vi "Lock VI.vi"(11 "文件路径":path) -> ()   [LabVIEW 2012]
panel:
  in  "密码":string="Jazz@0422g"
  out "滑动杆":i32(slide) scale=0.0..50.0
  out "All Files in Dir":path[](array[path]) caption="目录中的所有文件"
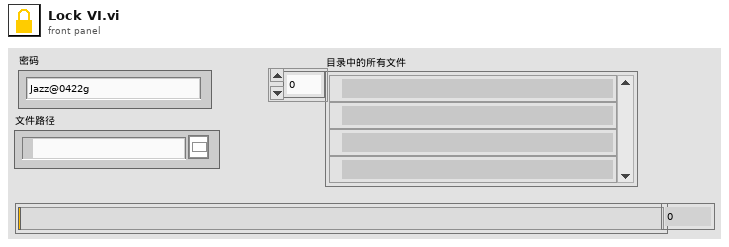
[diagram p1: front panel]
types:
  T1 = enum32{"invalid lock state", "Not Locked", "Locked (No Password)", "Password-protected"}
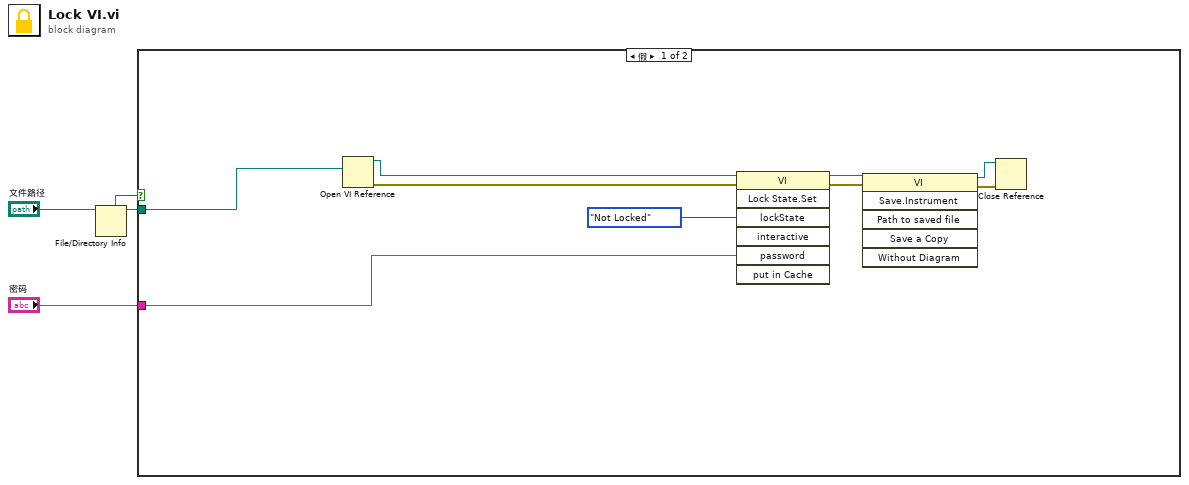
[diagram p0: block diagram]
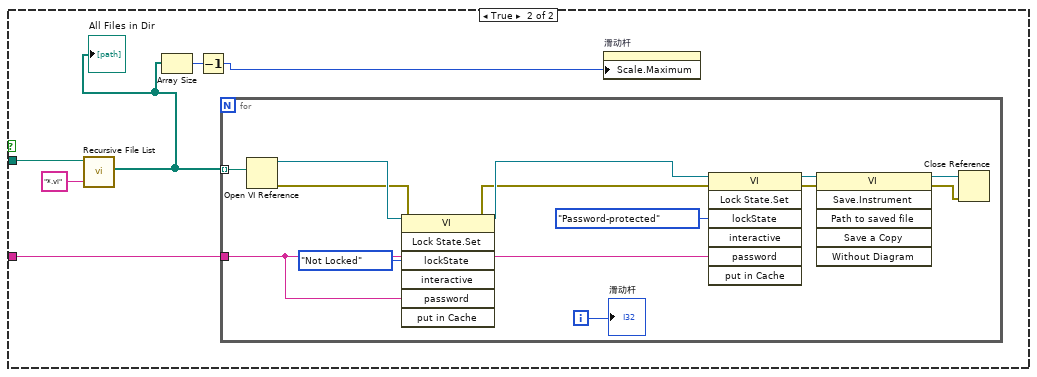
[diagram p2: hidden frame]
diagram:
  n1 = File/Directory Info(path="文件路径") -> (path out=w2:path, directory=w3:bool)  [unwired: 1 in, 5 out]
  n2 = case shown="假" w3 {
    tunnel: w2 -> [w10 w16]
    tunnel: "密码" -> [w5 w15]
    frame False {
      n3 = Open VI Reference(vi path=w10) -> (vi reference=w13:refnum<vi>, error out=w12:errorcluster)  [unwired: 5 in]
      n4 = invoke class="VI" method="Lock State.Set"(reference=w13, error in=w12, "lockState"=T1."Not Locked" ("锁定状态"), "password"=w5) -> (reference out=w8:refnum<vi>, error out=w9:errorcluster)  [unwired: 3 in, 5 out]
      n5 = invoke class="VI" method="Save.Instrument"(reference=w8, error in=w9) -> (reference out=w7:refnum<vi>, error out=w6:errorcluster)  [unwired: 4 in, 4 out]
      n6 = Close Reference(reference=w7, error in (no error)=w6) -> ()  [unwired: 1 out]
    }
    frame True {
      n7 = call <vilib>:"Recursive File List.vi"("pattern"="*.vi", "Folder Path"=w16) -> ("All Files in Dir"=w14:path[])  [unwired: 5 in, 4 out]
      "All Files in Dir" <- w14
      n8 = Array Size(array=w14) -> (size(s)=w18:i32)
      n9 = Decrement(x=w18) -> (x-1=w17:i32)
      n10 = for {
        tunnel: w14 -> [w31] mode=indexing
        tunnel: w15 -> [w20]
        i -> [w26]
        n11 = Open VI Reference(vi path=w31) -> (vi reference=w25:refnum<vi>, error out=w21:errorcluster)  [unwired: 5 in]
        n12 = invoke class="VI" method="Lock State.Set"(reference=w25, error in=w21, "lockState"=T1."Not Locked" ("锁定状态"), "password"=w20) -> (reference out=w24:refnum<vi>, error out=w22:errorcluster)  [unwired: 3 in, 5 out]
        n13 = invoke class="VI" method="Lock State.Set"(reference=w24, error in=w22, "lockState"=T1."Password-protected" ("锁定状态"), "password"=w20) -> (reference out=w30:refnum<vi>, error out=w27:errorcluster)  [unwired: 3 in, 5 out]
        n14 = invoke class="VI" method="Save.Instrument"(reference=w30, error in=w27) -> (reference out=w29:refnum<vi>, error out=w28:errorcluster)  [unwired: 4 in, 4 out]
        n15 = Close Reference(reference=w29, error in (no error)=w28) -> ()  [unwired: 1 out]
        "滑动杆" <- w26
      }
      n16 = property on="滑动杆" class="Slide (严格)"("Scale.Maximum"=w17) -> ()  [unwired: 2 in, 2 out]
    }
  }
